vi "Robot Global Data.vi"() -> ()   [LabVIEW 2015]
doc: "This global VI can contain as many global variables as you need. Place a control on the panel, give it a good name. To read or write to it from a VI, drag the icon to the diagram of that VI. You can also drag from the project. Click on the node to change which global you access. You shouldn't have multiple locations writing to a global or it will cause a race-condition."
uses:
  <vilib>/Rock Robotics/WPI/Camera/WPI_CameraImageSize.ctl
  <vilib>/Rock Robotics/WPI/DriverStation/WPI_DriverStationRobotMode2.ctl
  Drivetrain/Drivetrain Status.ctl
  Drivetrain/Drivetrain Commands.ctl
  Drivetrain/Drivetrain Modes.ctl
panel:
  in  "Drivetrain Command Cluster":T1
  out "Drivetrain Status Cluster":T3
  out "Gyro Roll Zero":dbl
  out "Gyro Pitch Zero":dbl
  out "Gyro Yaw Zero":dbl
  in  "Robot Mode":T4
  in  "image size":T5=enum."320x240"
  in  "Enable Vision":bool
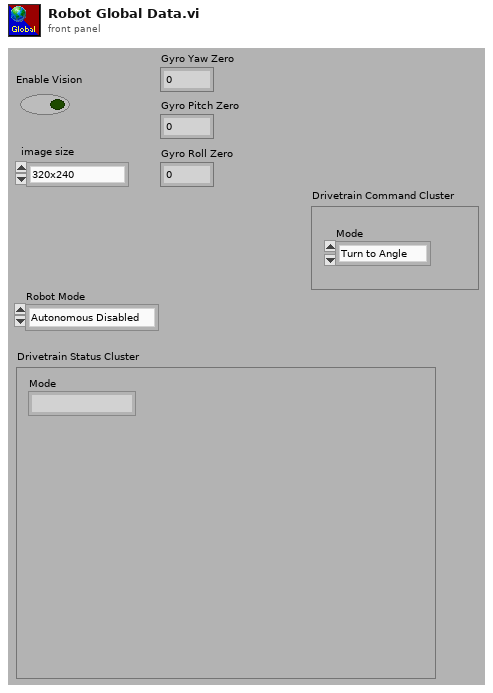
[diagram p1: front panel]
types:
  T1 = typedef "Drivetrain Commands.ctl" = cluster{"Mode":T2}
  T2 = typedef "Drivetrain Modes.ctl" = enum16{"Turn to Angle", "Distance Drive", "Data Acquisition", "Normal"}
  T3 = typedef "Drivetrain Status.ctl" = cluster{"Mode":enum16{""}}
  T4 = typedef "WPI_DriverStationRobotMode2.ctl" = enum16{"Autonomous Disabled", "Autonomous Enabled", "Teleop Disabled", "Teleop Enabled", "Disconnected", "Finish", "Test Disabled", "Test Enabled", "Emergency Stopped"}
  T5 = typedef "WPI_CameraImageSize.ctl" = enum16{"640x480", "320x240", "160x120", "Custom"}
diagram:
